vi "ATSh_GetSetParameterUL.vi"(0 "Handle":u32, 1 "Get / Set&Get":bool, 5 "Channel":u8, 7 "Parameter":u32 format="%08x", 9 "Value":u32) -> (4 "Handle_Out":u32, 10 "Value_Out":u32, 15 "Return Code":u32)   [LabVIEW 2014]
doc: "_____AlazarTech, Scope_____\n\nGet or Set parameter of the device.\nHandle as input."
uses:
  ATSApi.dll
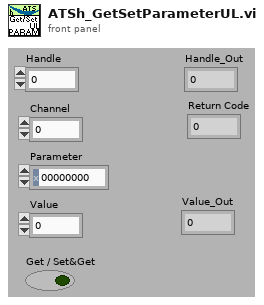
[diagram p1: front panel]
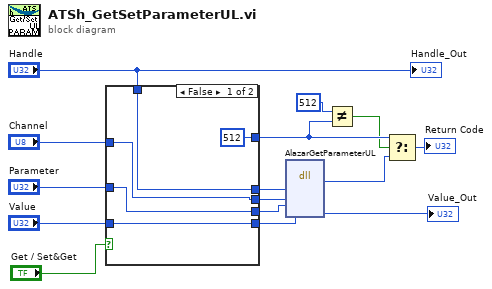
[diagram p0: block diagram]
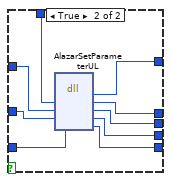
[diagram p2: hidden frame]
diagram:
  n1 = case shown="False" "Get / Set&Get" {
    tunnel: [u32 512 w29] -> w3
    tunnel: "Handle" -> [w20 w28]
    tunnel: "Value" -> [w18 w27]
    tunnel: [w18 w26] -> w12
    tunnel: [w20 w25] -> w11
    tunnel: "Parameter" -> [w16 w24]
    tunnel: "Channel" -> [w17 w23]
    tunnel: [w17 w22] -> w7
    tunnel: [w16 w21] -> w6
    frame False {
    }
    frame True {
      n2 = dll-call lib="D:/IntensityOCT/trunk/ATSApi.dll" fn="AlazarSetParameterUL" label="SetParameterUL"("Handle"=w28, "Channel"=w23, "Parameter"=w24, "Value"=w27) -> (w29:u32, "Handle"=w25:u32, "Channel"=w22:u8, "Parameter"=w21:u32, "Value"=w26:u32)  [unwired: 3 in, 2 out]
    }
  }
  n3 = dll-call lib="D:/IntensityOCT/trunk/ATSApi.dll" fn="AlazarGetParameterUL" label="GetParameterUL"("Handle"=w11, "Channel"=w7, "Parameter"=w6, "Value"=w12) -> (w5:u32, "Value"=→"Value_Out":u32)  [unwired: 6 in, 2 out]
  n4 = Not Equal?(x=u32 512, y=w3) -> (x != y?=w1:bool)
  n5 = Select(t=w3, s=w1, f=w5) -> (s? t:f=→"Return Code":u32)
  "Handle_Out" <- "Handle"
